vi "Configure Network Signaled Value.vi"(8 "error in (no error)":errorcluster, 9 "Network Signaled Value (NS01)":i32(ring)=1 items=["NS01"=1, "NS02"=2, "NS03"=3, "NS04"=4, "NS05"=5, "NS06"=6, "NS07"=7, "NS08"=8, "NS09"=9, "NS10"=10, "NS11"=11, "NS12"=12, "NS13"=13, "NS14"=14, "NS15"=15, "NS16"=16, "NS17"=17, "NS18"=18, "NS19"=19, "NS20"=20, "NS21"=21, "NS22"=22, "NS23"=23, "NS24"=24, "NS25"=25, "NS26"=26, "NS27"=27, "NS28"=28, "NS29"=29, "NS30"=30, "NS31"=31, "NS32"=32, "NS35"=35], 10 "Instance (1)":T1=1, 11 "VISA resource name":refnum<visa-resource-name>) -> (0 "error out":errorcluster, 3 "VISA resource name out":refnum<visa-resource-name>)   [LabVIEW 2020, in "Rohde&Schwarz CMWXP NR FR1 Measurement.lvlib"]
doc: "Selects the 'network signaled value'.\n\nAttribute:\nRSCMWXPNRFR1M_ATTR_NETWORK_SIGNALED_VALUE\n\nRemote-control command:\nCONFigure:NRSub:MEAS<i>:MEValuation:NSValue"
uses:
  <instrlib>/Rohde&Schwarz CMWXP NR FR1 Measurement/Rohde&Schwarz CMWXP NR FR1 Measurement.lvlib
  <instrlib>/Rohde&Schwarz CMWXP NR FR1 Measurement/Private/_Instance.ctl
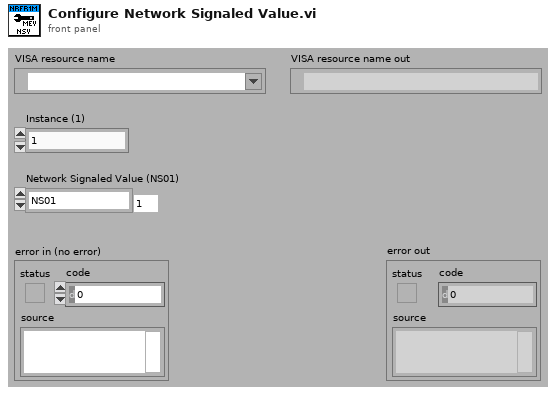
[diagram p1: front panel]
types:
  T1 = typedef "Rohde&Schwarz CMWXP NR FR1 Measurement.lvlib/_Instance.ctl" = i32
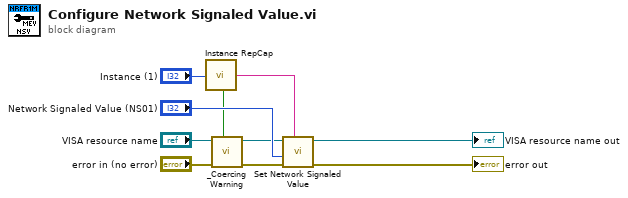
[diagram p0: block diagram]
diagram:
  n1 = call <instrlib>:"Instance RepCap.vi"("Instance In"="Instance (1)") -> ("In Range?"=w5:bool, "RepCap Identifier Out"=w6:string)  [unwired: 1 in]
  n2 = call <instrlib>:"_Coercing Warning.vi"("In Range?"=w5, "error in (no error)"="error in (no error)", "VISA resource name"="VISA resource name") -> ("error out"=w2:errorcluster, "VISA resource name out"=w1:refnum<visa-resource-name>)  [unwired: 7 in]
  n3 = call "Set Network Signaled Value"("Repeated Capabilities"=w6, "error in (no error)"=w2, "Network Signaled Value (1 - NS01)"="Network Signaled Value (NS01)", "instrument handle"=w1) -> ("error out"=→"error out":errorcluster, "instrument handle out"=→"VISA resource name out":refnum<visa-resource-name>)  [unwired: 6 in]
